vi "FileIO_FindPathByName.vi"(0 "Path In":path, 5 "File or Folder ?":enum16{"Folder", "File"}(ring)=enum."File", 7 "File/Folder Search String":string, 11 "Error In":errorcluster) -> (4 "Path Out":path, 6 "Found ?":bool, 8 "Report Text":string, 15 "Error Out":errorcluster)   [LabVIEW 2023]
doc: "This VI will search for a file/folder by name and return its path from within a given folder. If file/folder is not found returns empty path. Search string for file/folder name must be unique, if not it will return path for first match alphabetically.\n\nAlso returns a boolean for whether or not file/folder is found, along with report text when not found."
uses:
  <vilib>/regexp/Match Regular Expression.xnode
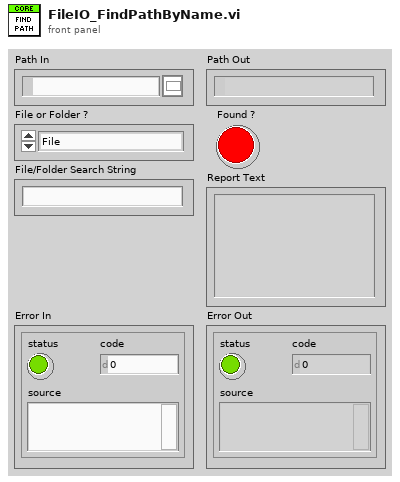
[diagram p1: front panel]
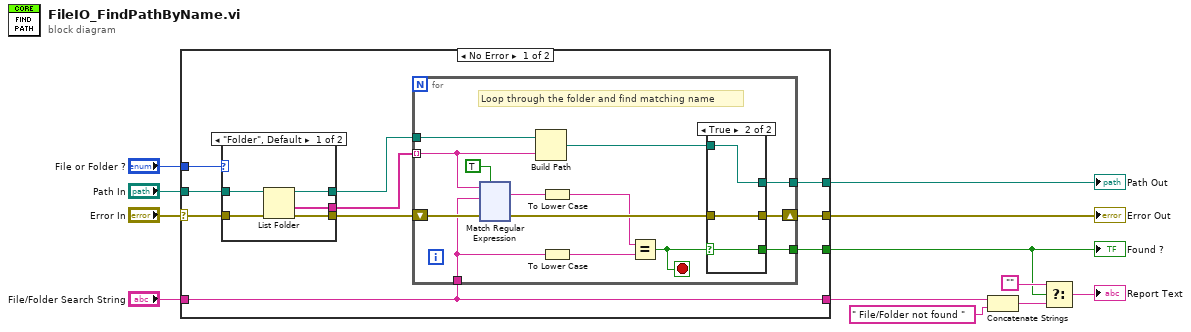
[diagram p0: block diagram]
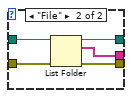
[diagram p2: hidden frame]
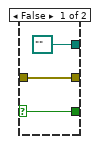
[diagram p3: hidden frame]
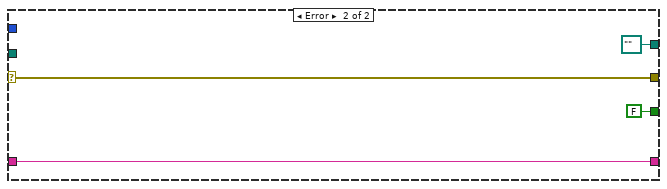
[diagram p4: hidden frame]
diagram:
  n1 = case shown="No Error" "Error In" {
    selector: "Error In" -> [w18 w173]
    tunnel: [w22 w173] -> w4
    tunnel: "Path In" -> [w19 _]
    tunnel: [w13 FALSE] -> w7
    tunnel: "File/Folder Search String" -> [w15 w172]
    tunnel: [w16 path "" ("appended path")] -> w1
    tunnel: "File or Folder ?" -> [w14 _]
    tunnel: [w15 w172] -> w9
    frame No Error {
      n2 = case shown="\"Folder\", Default" w14 {
        tunnel: [w23 w28] -> w21
        tunnel: [w26 w32] -> w20
        tunnel: w19 -> [w27 w31]
        tunnel: w18 -> [w25 w30]
        tunnel: [w24 w29] -> w17
        frame "Folder", Default {
          n3 = List Folder(path=w27, error in=w25) -> (path out=w26:path, folder names=w23:string[], error out=w24:errorcluster)  [unwired: 2 in, 1 out]
        }
        frame "File" {
          n4 = List Folder(path=w31, error in=w30) -> (path out=w32:path, filenames=w28:string[], error out=w29:errorcluster)  [unwired: 2 in, 1 out]
        }
      }
      n5 = for {
        shift-right: [w35] -> w22
        shift-left: w17 -> [w44]
        tunnel: w21 -> [w42] mode=indexing
        tunnel: w20 -> [w45]
        tunnel: w15 -> [w40]
        tunnel: [w41] -> w16
        tunnel: [w38] -> w13
        stop <- w37 stop-if-true
        # "Loop through the folder and find matching name"
        n6 = xnode "Match Regular Expression"("input string"=w42, "regular expression"=w40, "error in"=w44, "ignore case? (F)"=TRUE) -> ("whole match"=w39:string, "error out"=w36:errorcluster)  [unwired: 2 in, 3 out]
        n7 = Build Path(base path=w45, name or relative path=w42) -> (appended path=w46:path)
        n8 = To Lower Case(string=w39) -> (all lower case string=w34:string)
        n9 = To Lower Case(string=w40) -> (all lower case string=w33:string)
        n10 = Equal?(x=w34, y=w33) -> (x = y?=w37:bool)
        n11 = case shown="True" w37 {
          selector: w37 -> [w164 w168]
          tunnel: w46 -> [_ w169]
          tunnel: [path "" w169] -> w41
          tunnel: [w164 w168] -> w38
          tunnel: w36 -> [w165 w167]
          tunnel: [w165 w167] -> w35
          frame False {
          }
          frame True {
          }
        }
      }
    }
    frame Error {
    }
  }
  "Found ?" <- w7
  "Error Out" <- w4
  "Path Out" <- w1
  n12 = Concatenate Strings(w9, " File/Folder not found ") -> (w6:string)
  n13 = Select(t="", s=w7, f=w6) -> (s? t:f=→"Report Text":string)
